vi "DC Voltage Get Range.vi"(8 "error in (no error)":errorcluster {"code" format="%.0x"}, 9 "ValBufferSize":i32=2048, 10 "ChannelList":string, 11 "instrument handle":refnum<k15>) -> (0 "error out":errorcluster {"code" format="%.0x"}, 1 "ValActualSize":i32, 2 "Val":dbl[](array[numeric]) format="%.2p", 3 "instrument handle out":refnum<k15>)   [LabVIEW 2020, in "Keysight DAQ970.lvlib"]
doc: "Gets the measurement range in volts of the specified channelList or current scan list if parameter is empty."
uses:
  Keysight DAQ970.lvlib
  KtDAQ970.dll
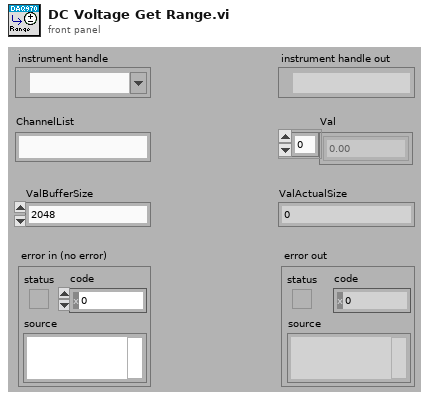
[diagram p1: front panel]
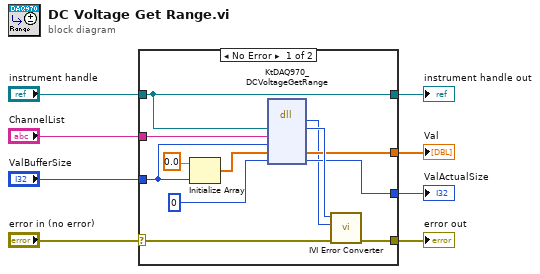
[diagram p0: block diagram]
diagram:
  n1 = case shown="No Error" "error in (no error)" {
    selector: "error in (no error)" -> [w19 w22]
    tunnel: [w18 w22] -> w8
    tunnel: "instrument handle" -> [w11 w21]
    tunnel: "ChannelList" -> [w17 _]
    tunnel: "ValBufferSize" -> [w10 _]
    tunnel: [w14 _] -> w3
    tunnel: [w12 _] -> w2
    tunnel: [w11 w21] -> w1
    frame No Error {
      n2 = Initialize Array(0.0 ("element"), w10) -> (w16:dbl[])
      n3 = dll-call lib="KtDAQ970**.dll" fn="KtDAQ970_DCVoltageGetRange"("Vi"=w11, "ChannelList"=w17, "ValBufferSize"=w10, "Val"=w16, "ValActualSize"=0) -> (w9:i32, "Vi"=w20:u32, "Val"=w14:dbl[], "ValActualSize"=w12:i32)  [unwired: 5 in, 2 out]
      n4 = call "IVI Error Converter.vi"("error in (no error)"=w19, "IVI error code (0)"=w9, "instrument handle"=w20) -> ("error out"=w18:errorcluster)  [unwired: 7 in, 1 out]
    }
    frame Error {
    }
  }
  "error out" <- w8
  "instrument handle out" <- w1
  "Val" <- w3
  "ValActualSize" <- w2
